vi "RunTimeMenu Custom Population.vi"(8 "error in":errorcluster, 10 "Menu Refnum":refnum<k9>, 11 "Node Ptr":u64 format="%.0x") -> (0 "error out":errorcluster)   [LabVIEW 2020, in "AIM MIL-STD-1553 System Explorer.lvlib"]
uses:
  AIM MIL-STD-1553 System Explorer.lvlib
  Includes/AIM MIL-STD-1553 System Explorer.lvlibp/System Explorer/Interfaces/System Explorer Dispatcher/System Explorer Dispatcher.lvclass
  Includes/AIM MIL-STD-1553 System Explorer.lvlibp/System Explorer/Implementation/System Explorer Dispatcher/System Explorer Dispatcher.lvclass
  C:/dev/git/niveristand-aim-milStd1553-custom-device/Includes/AIM MIL-STD-1553 System Explorer.lvlibp/System Explorer/Interfaces/System Explorer Dispatcher/System Explorer Dispatcher.lvclass
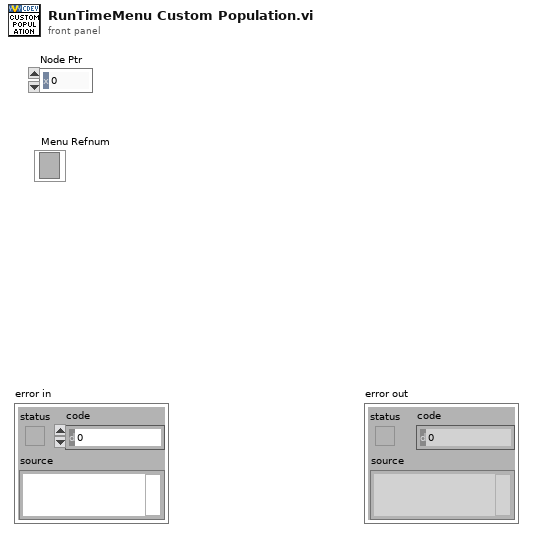
[diagram p1: front panel]
types:
  T1 = typedef "Custom Device API.lvlib/Custom Device Item Ref.ctl" = u64
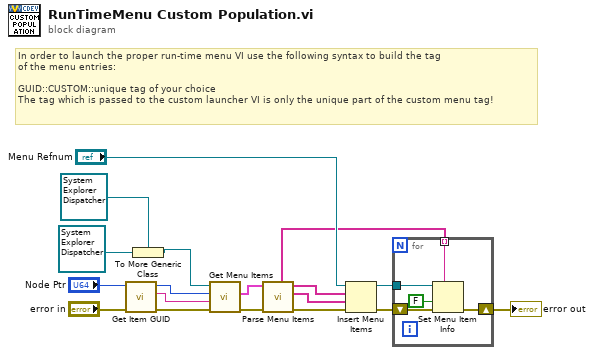
[diagram p0: block diagram]
diagram:
  # "In order to launch the proper run-time menu VI use the following syntax to build the tag\nof the menu entries:\n\nGUID::CUSTOM::unique tag of your choice\nThe tag which is passed to the custom launcher VI is only the unique part of the custom menu tag!"
  n1 = call "Get Item GUID.vi"("error in (no error)"="error in", "item in"="Node Ptr") -> ("error out"=w9:errorcluster, "guid"=w8:string, "item out"=w7:T1)  [unwired: 7 in]
  n2 = To More Generic Class(target class=refnum<class "System Explorer Dispatcher.lvclass"> refnum ("AIM MIL-STD-1553 System Explorer.lvlibp:Interfaces.lvlib:System Explorer Dispatcher.lvclass"), reference=refnum<class "System Explorer Dispatcher.lvclass"> refnum ("AIM MIL-STD-1553 System Explorer.lvlibp:Implementation.lvlib:System Explorer Dispatcher.lvclass")) -> (generic class reference=w12:refnum<class "System Explorer Dispatcher.lvclass">)
  n3 = call-dynamic "Get Menu Items.vi"("error in (no error)"=w9, "GUID"=w8, "Item Ref"=w7, "System Explorer Dispatcher in"=w12) -> ("error out"=w2:errorcluster, "Menu Items"=w1:cluster{"Name":string, "Enabled?":bool}[])  [unwired: 5 in, 1 out]
  n4 = call "Parse Menu Items.vi"("error in"=w2, "Menu Items"=w1) -> ("error out"=w3:errorcluster, "Item Tags"=w4:string[], "Item Names"=w5:string[], "Disabled Tags"=w6:string[])  [unwired: 6 in]
  n5 = Insert Menu Items(6:w3, 7:w4, 8:w5, 9:"Menu Refnum") -> (0:w16:errorcluster, 3:w17:refnum<k9>)  [unwired: 2 in, 1 out]
  n6 = for {
    tunnel: w17 -> [w23]
    shift-right: [w21] -> w15
    shift-left: w16 -> [w22]
    tunnel: w6 -> [w19] mode=indexing
    n7 = Set Menu Item Info(7:w19, 8:w22, 9:FALSE ("enabled"), 11:w23) -> (0:w21:errorcluster)  [unwired: 3 in, 1 out]
  }
  "error out" <- w15
